vi "Display Module Check and Run.vi"() -> (8 "Error":errorcluster)   [LabVIEW 2016]
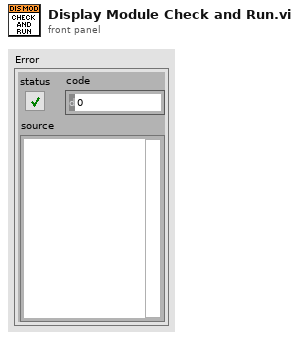
[diagram p1: front panel]
types:
  T1 = enum32{"Bad", "Idle", "Run top level", "Running"}
  T2 = enum32{"Invalid", "Standard", "Closed", "Hidden", "Minimized", "Maximized"}
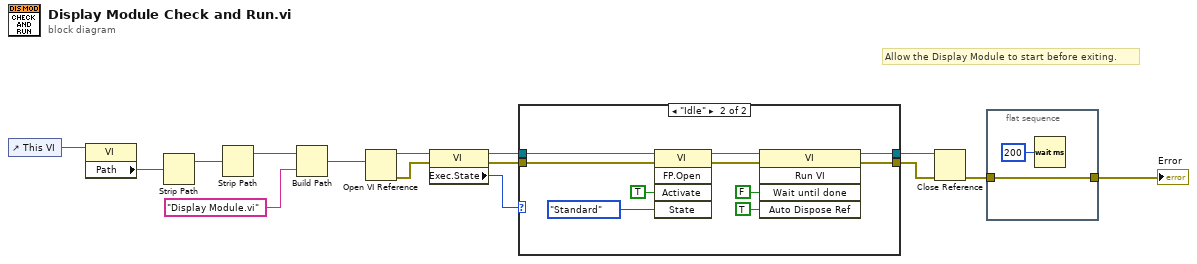
[diagram p0: block diagram]
diagram:
  # "Allow the Display Module to start before exiting."
  n1 = control-ref of="This VI"() -> (w15:refnum<vi>)
  n2 = property class="VI"(reference=w15) -> ("Path"=w14:path)  [unwired: 1 in, 2 out]
  n3 = Strip Path(path=w14) -> (stripped path=w13:path)  [unwired: 1 out]
  n4 = Strip Path(path=w13) -> (stripped path=w12:path)  [unwired: 1 out]
  n5 = Build Path(base path=w12, name or relative path="Display Module.vi") -> (appended path=w8:path)
  n6 = Open VI Reference(vi path=w8) -> (vi reference=w10:refnum<vi>, error out=w7:errorcluster)  [unwired: 5 in]
  n7 = property class="VI"(reference=w10, error in=w7) -> (reference out=w6:refnum<vi>, error out=w5:errorcluster, "Exec.State"=w9:T1)
  n8 = case shown="\"Idle\"" w9 {
    tunnel: w5 -> [w17 w21]
    tunnel: [w17 w19] -> w3
    tunnel: w6 -> [w16 w22]
    tunnel: [w16 w18] -> w4
    frame Default {
    }
    frame "Idle" {
      n9 = invoke class="VI" method="FP.Open"(reference=w22, error in=w21, "Activate"=TRUE ("Activate?"), "State"=T2."Standard") -> (reference out=w25:refnum<vi>, error out=w20:errorcluster)  [unwired: 1 in, 3 out]
      n10 = invoke class="VI" method="Run VI"(reference=w25, error in=w20, "Wait until done"=FALSE ("Wait Until Done"), "Auto Dispose Ref"=TRUE ("Auto Dispose Reference")) -> (reference out=w18:refnum<vi>, error out=w19:errorcluster)  [unwired: 1 in, 3 out]
    }
  }
  n11 = Close Reference(reference=w4, error in (no error)=w3) -> (error out=w2:errorcluster)
  n12 = flat-sequence {
    tunnel: [w29] -> w1
    tunnel: w2 -> [w29]
    frame #0 {
      n13 = Wait (ms)(milliseconds to wait=u32 200) -> ()  [unwired: 1 out]
    }
  }
  "Error" <- w1
